vi "Post-Uninstall Custom Action.vi"(10 "Variant":variant) -> (0 "error out":errorcluster)   [LabVIEW 2024]
uses:
  <vilib>/Utility/error.llb/Trim Whitespace One-Sided.vi
  <vilib>/Utility/file.llb/Read Delimited Spreadsheet (string).vi
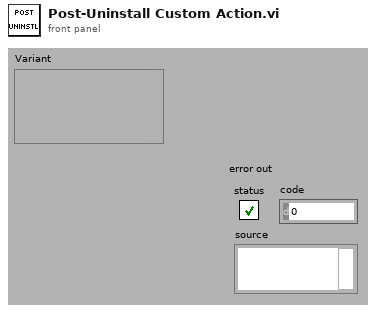
[diagram p1: front panel]
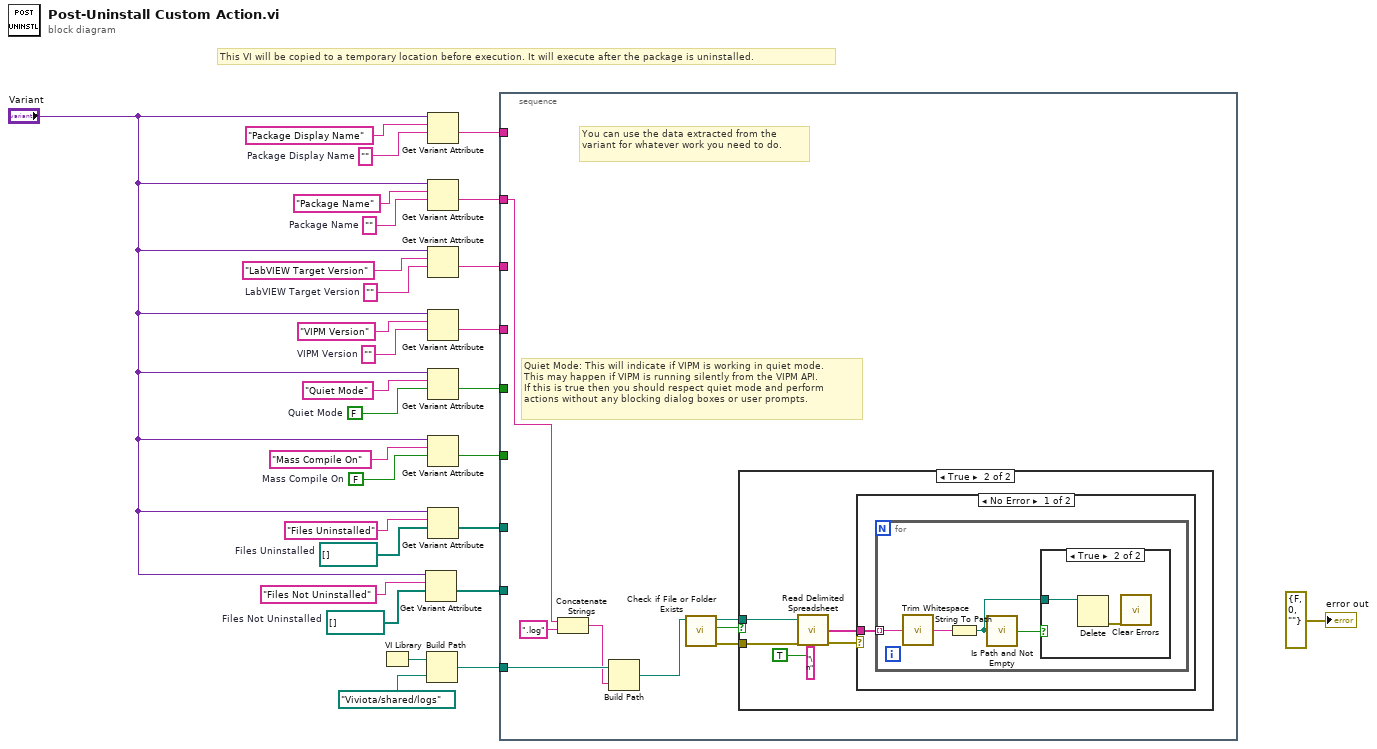
[diagram p0: block diagram]
diagram:
  w4 = path[] []  # Files Not Uninstalled
  w5 = path[] []  # Files Uninstalled
  w11 = FALSE  # Mass Compile On
  w12 = ""  # Package Display Name
  w19 = FALSE  # Quiet Mode
  w22 = ""  # VIPM Version
  w24 = ""  # LabVIEW Target Version
  w26 = ""  # Package Name
  # "This VI will be copied to a temporary location before execution. It will execute after the package is uninstalled."
  n1 = VI Library() -> (path=w3:path)
  n2 = Get Variant Attribute(Variant="Variant", name="Files Not Uninstalled", default value (empty Variant)=w4) -> (value=w9:path[])  [unwired: 1 in, 3 out]
  n3 = Build Path(base path=w3, name or relative path=path "Viviota/shared/logs") -> (appended path=w1:path)
  n4 = Get Variant Attribute(Variant="Variant", name="Package Display Name", default value (empty Variant)=w12) -> (value=w18:string)  [unwired: 1 in, 3 out]
  n5 = Get Variant Attribute(Variant="Variant", name="Package Name", default value (empty Variant)=w26) -> (value=w17:string)  [unwired: 1 in, 3 out]
  n6 = Get Variant Attribute(Variant="Variant", name="LabVIEW Target Version", default value (empty Variant)=w24) -> (value=w16:string)  [unwired: 1 in, 3 out]
  n7 = Get Variant Attribute(Variant="Variant", name="VIPM Version", default value (empty Variant)=w22) -> (value=w15:string)  [unwired: 1 in, 3 out]
  n8 = Get Variant Attribute(Variant="Variant", name="Quiet Mode", default value (empty Variant)=w19) -> (value=w14:bool)  [unwired: 1 in, 3 out]
  n9 = Get Variant Attribute(Variant="Variant", name="Mass Compile On", default value (empty Variant)=w11) -> (value=w13:bool)  [unwired: 1 in, 3 out]
  n10 = Get Variant Attribute(Variant="Variant", name="Files Uninstalled", default value (empty Variant)=w5) -> (value=w8:path[])  [unwired: 1 in, 3 out]
  n11 = stacked-sequence {
    tunnel: w18 -> [_]
    tunnel: w17 -> [w31]
    tunnel: w16 -> [_]
    tunnel: w15 -> [_]
    tunnel: w14 -> [_]
    tunnel: w13 -> [_]
    tunnel: w8 -> [_]
    tunnel: w9 -> [_]
    tunnel: w1 -> [w36]
    frame #0 {
      # "Quiet Mode: This will indicate if VIPM is working in quiet mode.\nThis may happen if VIPM is running silently from the VIPM API.\nIf this is true then you should respect quiet mode and perform\nactions without any blocking dialog boxes or user prompts."
      # "You can use the data extracted from the variant for whatever work you need to do."
      n12 = Concatenate Strings(w31, ".log" ("string")) -> (w35:string)
      n13 = Build Path(base path=w36, name or relative path=w35) -> (appended path=w30:path)
      n14 = call <vilib>:"Check if File or Folder Exists.vi"("path"=w30) -> ("error out"=w32:errorcluster, "file or folder exists?"=w34:bool, "dup path"=w33:path)  [unwired: 8 in]
      n15 = case shown="True" w34 {
        tunnel: w33 -> [_ w43]
        tunnel: w32 -> [_ w40]
        frame False {
        }
        frame True {
          n16 = call-poly <vilib>:"Read Delimited Spreadsheet.vi"("file path (dialog if empty)"=w43, "error in (no error)"=w40, "transpose? (F)"=TRUE, "delimiter (\\t)"="\n" ("delimiter (\\t)")) -> ("first row"=w41:string[], "error out"=w39:errorcluster)  [unwired: 6 in, 4 out]
          n17 = case shown="No Error" w39 {
            tunnel: w41 -> [w44 _]
            frame No Error {
              n18 = for {
                tunnel: w44 -> [w48] mode=indexing
                n19 = call <vilib>:"Trim Whitespace.vi"("string"=w48) -> ("trimmed string"=w47:string)  [unwired: 1 in]
                n20 = String To Path(string=w47) -> (path=w45:path)
                n21 = call <vilib>:"Is Path and Not Empty.vi"("path"=w45) -> ("Is Path and Not Empty?"=w46:bool)  [unwired: 4 in]
                n22 = case shown="True" w46 {
                  tunnel: w45 -> [_ w50]
                  frame False {
                  }
                  frame True {
                    n23 = Delete(path (use dialog)=w50) -> (error out=w49:errorcluster)  [unwired: 4 in, 2 out]
                    n24 = call <vilib>:"Clear Errors.vi"("error in (no error)"=w49) -> ()  [unwired: 5 in, 2 out]
                  }
                }
              }
            }
            frame Error {
            }
          }
        }
      }
    }
  }
  "error out" <- errorcluster {"status"=FALSE, "code"=0, "source"=""} ("error out")
